vi "sourcemeter and multimeter.vi"() -> ()   [LabVIEW 2018]
panel:
  in  "String 2":string="v_dn_21July.lvm"
  in  "String1":string="N_2205_pressure_"
  in  "File Save Folder":path=path "D:/Soumen/OrbitalShaker/Pressure measurement/2205 particles/Run_21July/heating"
  in  "File save - yes/ no?":bool
  in  "For loop count":i32=1000
  in  "Direction - up (on)/ down(off)":bool=TRUE
  in  "format string":string="%0.2f"
  in  "Step":dbl
  in  "End Voltage":dbl
  in  "Start Voltage":dbl
  out "Save File Path":path
  out "Reading Result":string
  out "error out":T1
  out "value":dbl
  out "Waveform Chart":dbl(graph)
  in  "error in":T1
  in  "stop":bool
  out "Measure loop":i32
  in  "function (Vdc:1)":u16(ring)=1 items=["ac voltage", "dc voltage", "2-wire resistance", "4-wire resistance", "ac current", "dc current", "frequency", "temperature"]
  in  "GPIB Address":string="16"
  out "Voltage Loop":i32
  out "Set Voltage":string
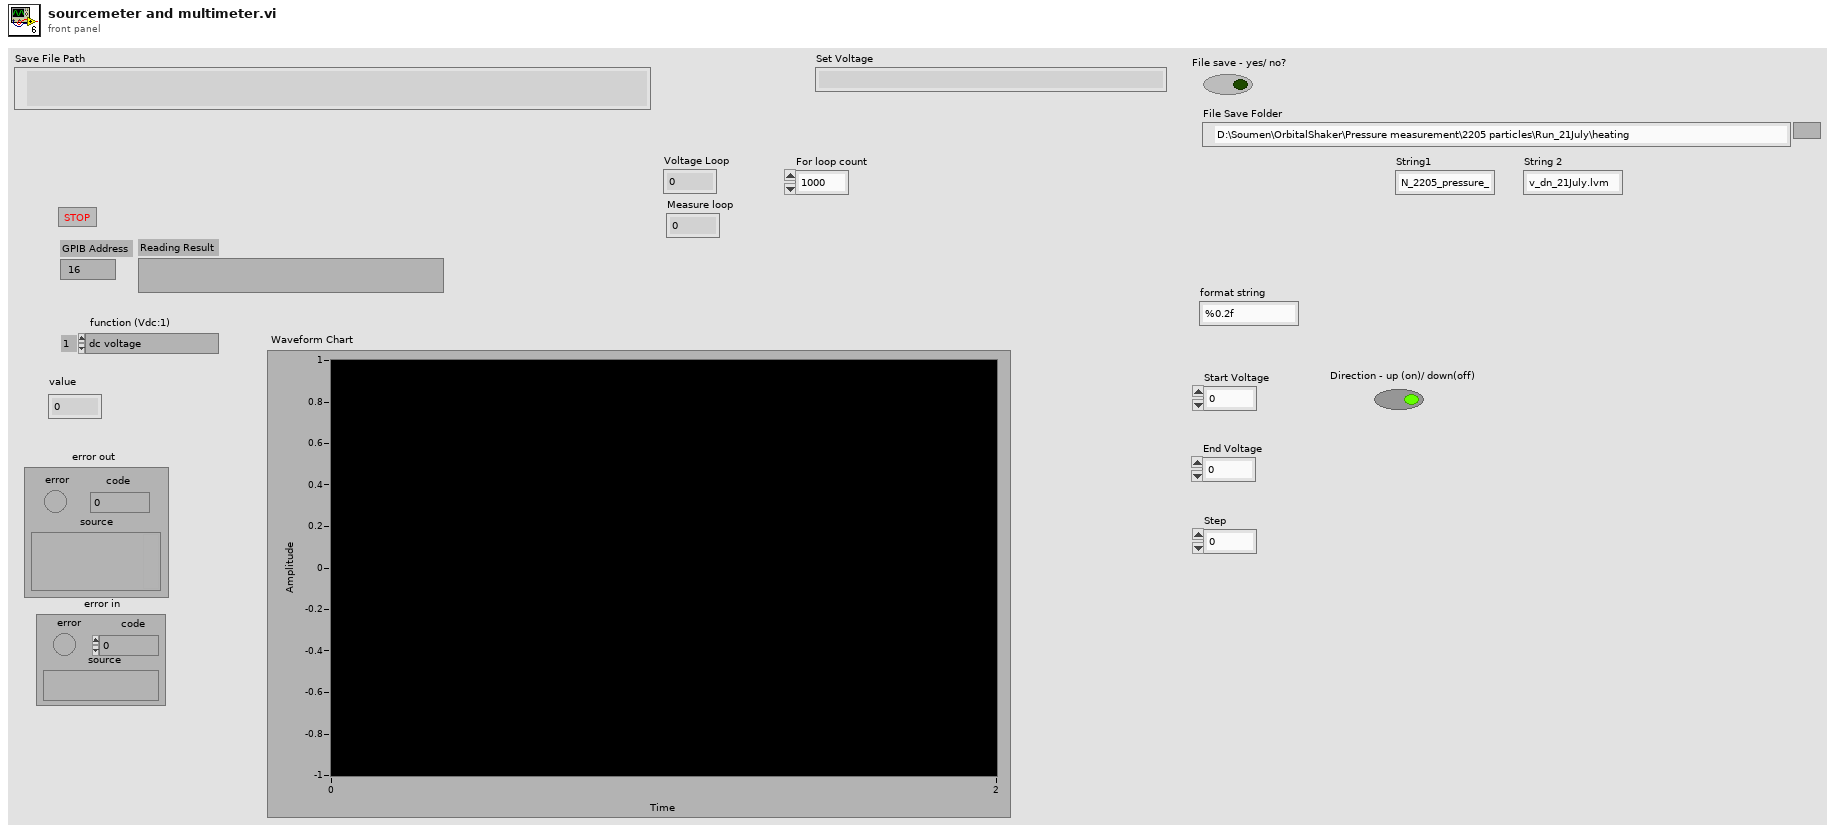
[diagram p1: front panel]
types:
  T1 = cluster{"error":bool, "code":i32, "source":string}
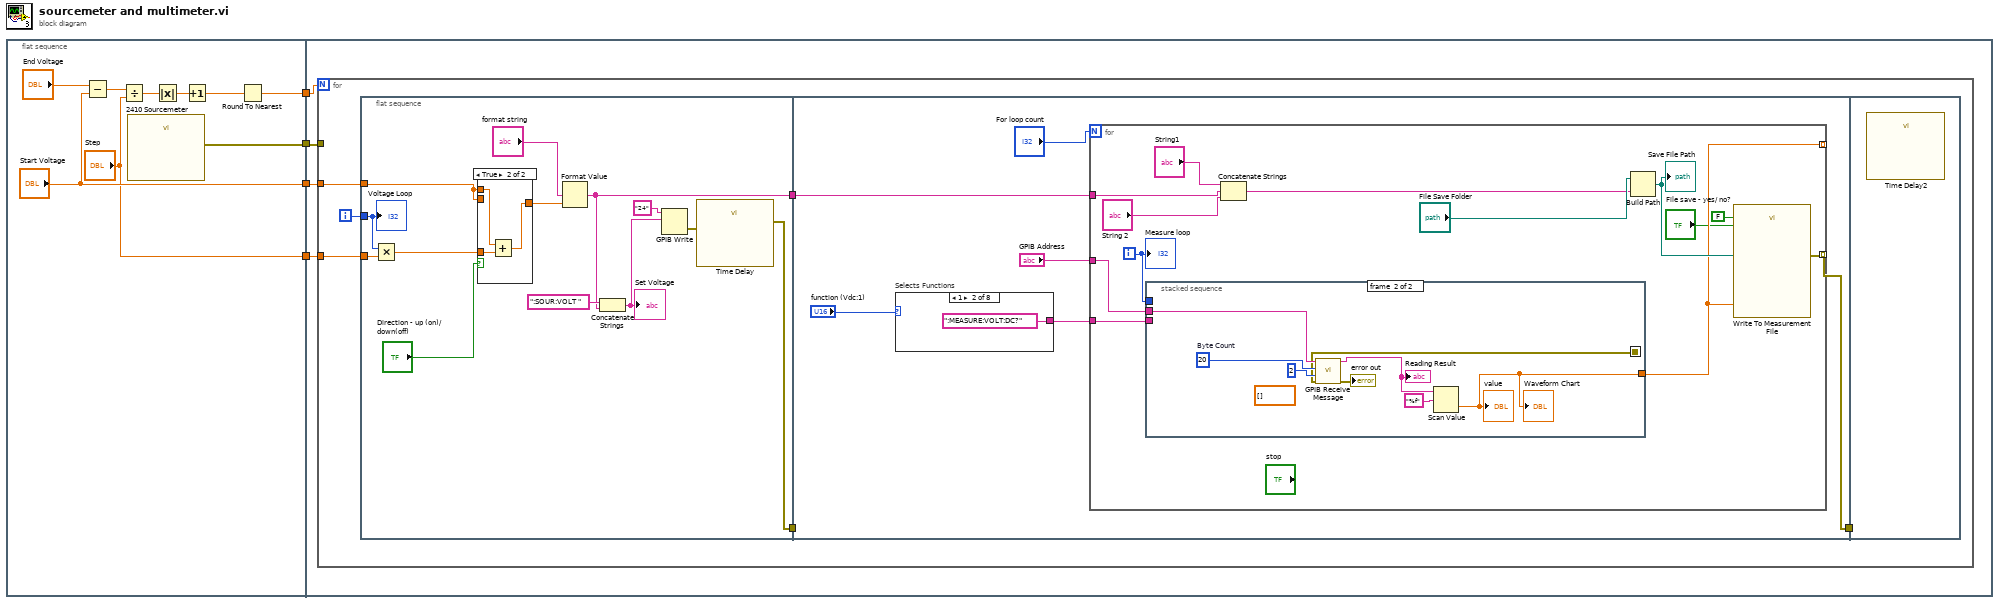
[diagram p0: block diagram]
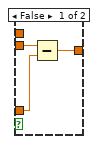
[diagram p2: hidden frame]
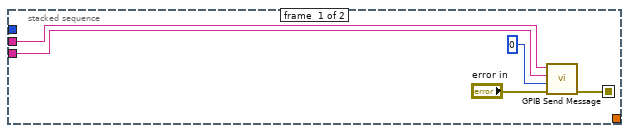
[diagram p3: hidden frame]
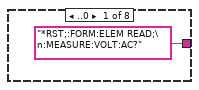
[diagram p4: hidden frame]
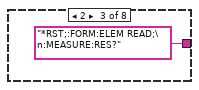
[diagram p5: hidden frame]
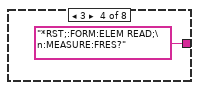
[diagram p6: hidden frame]
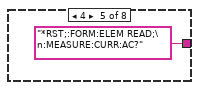
[diagram p7: hidden frame]
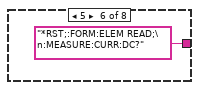
[diagram p8: hidden frame]
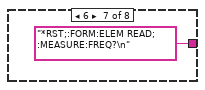
[diagram p9: hidden frame]
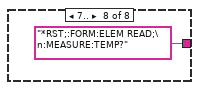
[diagram p10: hidden frame]
diagram:
  n1 = flat-sequence {
    tunnel: [w10] -> w4
    tunnel: ["Start Voltage"] -> w3
    tunnel: ["Step"] -> w2
    tunnel: [w5] -> w1
    tunnel: w4 -> [w17]
    tunnel: w3 -> [w16]
    tunnel: w2 -> [w15]
    tunnel: w1 -> [w14]
    frame #0 {
      n2 = Subtract(x="End Voltage", y="Start Voltage") -> (x-y=w12:dbl)
      n3 = Divide(x=w12, y="Step") -> (x/y=w7:dbl)
      n4 = call "2410 Sourcemeter"() -> ("error out"=w5:errorcluster)  [unwired: 26 in, 1 out]
      n5 = Absolute Value(x=w7) -> (abs(x)=w6:dbl)
      n6 = Increment(x=w6) -> (x+1=w11:dbl)
      n7 = Round To Nearest(number=w11) -> (nearest integer value=w10:dbl)
    }
    frame #1 {
      n8 = for {
        N: w17 -> [_]
        tunnel: w16 -> [w19]
        tunnel: w15 -> [w18]
        tunnel: w14 -> [_]
        i -> [w23]
        n9 = flat-sequence {
          tunnel: w23 -> [w28]
          tunnel: [w32] -> w22
          tunnel: [w30] -> w20
          tunnel: w19 -> [w24]
          tunnel: w18 -> [w29]
          tunnel: w22 -> [_]
          tunnel: [w44] -> w21
          tunnel: w20 -> [w43]
          tunnel: w21 -> [_]
          frame #0 {
            n10 = Multiply(x=w28, y=w29) -> (x*y=w27:dbl)
            n11 = case shown="True" "Direction - up (on)/ down(off)" {
              tunnel: w27 -> [w38 w42]
              tunnel: w24 -> [_ w41]
              tunnel: [w39 w40] -> w25
              tunnel: w24 -> [w37 _]
              frame False {
                n12 = Subtract(x=w37, y=w38) -> (x-y=w39:dbl)
              }
              frame True {
                n13 = Add(x=w41, y=w42) -> (x+y=w40:dbl)
              }
            }
            n14 = Format Value(format string="format string", value (0)=w25) -> (output string=w30:string)  [unwired: 1 in]
            n15 = Concatenate Strings(":SOUR:VOLT ", w30) -> (w31:string)
            "Set Voltage" <- w31
            n16 = GPIB Write(0:"24" ("address string"), 1:w31) -> (6:w33:errorcluster)  [unwired: 3 in, 1 out]
            n17 = call "Time Delay"("error in (no error)"=w33) -> ("error out"=w32:errorcluster)  [unwired: 10 in]
            "Voltage Loop" <- w28
          }
          frame #1 {
            n18 = case "Selects Functions" shown="1" "function (Vdc:1)" {
              tunnel: ["*RST;:FORM:ELEM READ;\n:MEASURE:VOLT:AC?" ":MEASURE:VOLT:DC?" "*RST;:FORM:ELEM READ;\n:MEASURE:RES?" "*RST;:FORM:ELEM READ;\n:MEASURE:FRES?" "*RST;:FORM:ELEM READ;\n:MEASURE:CURR:AC?" "*RST;:FORM:ELEM READ;\n:MEASURE:CURR:DC?" "*RST;:FORM:ELEM READ; :MEASURE:FREQ?\n" "*RST;:FORM:ELEM READ;\n:MEASURE:TEMP?"] -> w46
              frame ..0 {
              }
              frame 1 {
              }
              frame 2 {
              }
              frame 3 {
              }
              frame 4 {
              }
              frame 5 {
              }
              frame 6 {
              }
              frame 7.. {
              }
            }
            n19 = for {
              N: "For loop count" -> [_]
              tunnel: "GPIB Address" -> [w61]
              tunnel: w46 -> [w60]
              tunnel: [w50] -> _ mode=indexing
              tunnel: [w58] -> w44 mode=indexing
              tunnel: w43 -> [w51]
              i -> [w59]
              n20 = stacked-sequence {
                seq-local: [w62 _] -> [_ w71]
                tunnel: w61 -> [w66 w74]
                tunnel: w60 -> [w63 _]
                tunnel: w59 -> [_ _]
                tunnel: [_ w67] -> w50
                frame #0 {
                  n21 = call "GPIB Send Message.vi"("address string"=w66, "write buffer"=w63, "write mode (set END:0)"=0, "error in"="error in") -> ("error out"=w62:T1)  [unwired: 3 in, 2 out]
                }
                frame #1 {
                  (unwired) dbl[] [] ("Waveform Graph")
                  w73 = 20  # Byte Count
                  n22 = call "GPIB Receive Message.vi"("address string"=w74, "byte count"=w73, "read mode"=2, "error in"=w71) -> ("read buffer"=w69:string, "error out"=→"error out":T1)  [unwired: 3 in, 1 out]
                  "Reading Result" <- w69
                  n23 = Scan Value(string=w69, format string="%f") -> (value=w67:dbl)  [unwired: 1 in, 1 out]
                  "value" <- w67
                  "Waveform Chart" <- w67
                }
              }
              n24 = Concatenate Strings("String1", w51, "String 2") -> (w54:string)
              n25 = Build Path(base path="File Save Folder", name or relative path=w54) -> (appended path=w53:path)
              "Save File Path" <- w53
              n26 = call "Write To Measurement File"("Signals"=w50, "Reset"=FALSE, "Enable"="File save - yes/ no?", "Filename"=w53) -> ("error out"=w58:errorcluster)  [unwired: 13 in, 2 out]
              "Measure loop" <- w59
            }
          }
          frame #2 {
            n27 = call "Time Delay2"() -> ()  [unwired: 11 in, 1 out]
          }
        }
      }
    }
  }
